vi "Rename Category.vi"(8 "error in (no error)":errorcluster, 9 "Name":string, 10 "Category in":refnum<class "Category.lvclass">, 11 "Database in":refnum<class "Account History.lvclass">) -> (0 "error out":errorcluster, 3 "Database out":refnum<class "Account History.lvclass">)   [LabVIEW 2018, in "Account History.lvclass"]
uses:
  Account History.lvclass
  Category/Category.lvclass
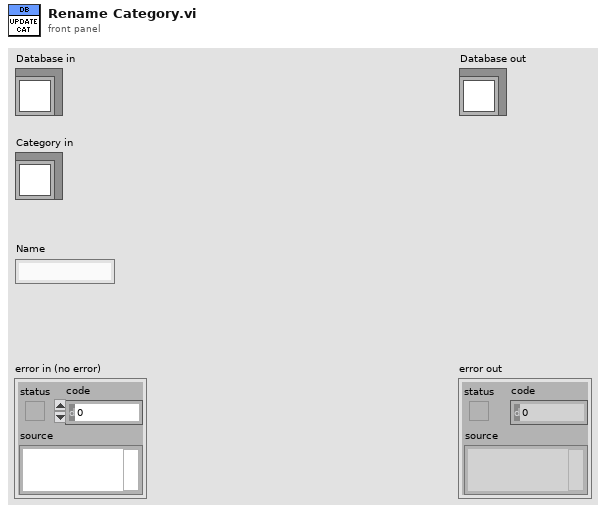
[diagram p1: front panel]
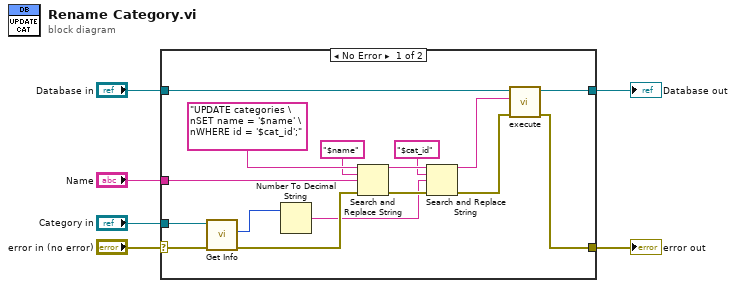
[diagram p0: block diagram]
diagram:
  n1 = case shown="No Error" "error in (no error)" {
    selector: "error in (no error)" -> [w18 w23]
    tunnel: "Database in" -> [w22 w24]
    tunnel: [w21 w24] -> w5
    tunnel: [w20 w23] -> w4
    tunnel: "Name" -> [w8 _]
    tunnel: "Category in" -> [w17 _]
    frame No Error {
      n2 = call "Get Info.vi"("error in (no error)"=w18, "Category in"=w17) -> ("error out"=w16:errorcluster, "id"=w19:i32)  [unwired: 6 in, 2 out]
      n3 = Number To Decimal String(number=w19) -> (decimal integer string=w7:string)  [unwired: 1 in]
      n4 = Search and Replace String(input string="UPDATE categories \nSET name = '$name' \nWHERE id = '$cat_id';", search string="$name", replace string=w8, error in=w16) -> (result string=w12:string, error out=w15:errorcluster)  [unwired: 4 in, 2 out]
      n5 = Search and Replace String(input string=w12, search string="$cat_id", replace string=w7, error in=w15) -> (result string=w11:string, error out=w14:errorcluster)  [unwired: 4 in, 2 out]
      n6 = call "execute.vi"("error in (no error)"=w14, "SQL query"=w11, "Database in"=w22) -> ("error out"=w20:errorcluster, "Database out"=w21:refnum<class "Account History.lvclass">)  [unwired: 7 in]
    }
    frame Error {
    }
  }
  "error out" <- w4
  "Database out" <- w5
